vi "BlueToothOff.vi"(4 "Connected":bool, 5 "Partner Name":string, 6 "Connection":u8, 7 "NXT/EV3":T1) -> (1 "Success":bool, 2 "NXTBTPower":i8, 3 "NXT/EV3 2":T1)   [LabVIEW 2013]
uses:
  <vilib>/NXT/Subs/LVHSConnector.ctl
  <vilib>/NXT/LegoClasses/BrickReference/BrickReference.lvclass
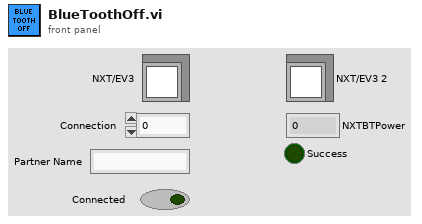
[diagram p1: front panel]
types:
  T1 = typedef "LVHSConnector.ctl" = refnum<class "BrickReference.lvclass">
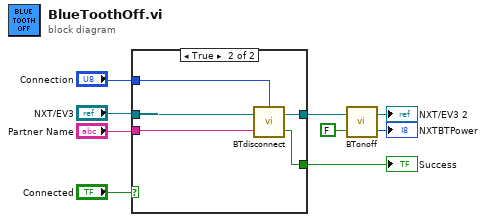
[diagram p0: block diagram]
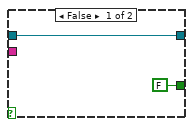
[diagram p2: hidden frame]
diagram:
  n1 = case shown="True" "Connected" {
    tunnel: "NXT/EV3" -> [w11 w16]
    tunnel: [w11 w15] -> w7
    tunnel: [FALSE ("Success") w14] -> w3
    tunnel: "Partner Name" -> [_ w13]
    tunnel: "Connection" -> [_ w12]
    frame False {
    }
    frame True {
      n2 = call <vilib>:"BTdisconnect.vi"("Partner Name"=w13, "NXT/EV3"=w16, "Connection"=w12) -> ("Success"=w14:bool, "NXT/EV3"=w15:T1)
    }
  }
  "Success" <- w3
  n3 = call <vilib>:"BTonoff.vi"("On/Off"=FALSE, "NXT/EV3"=w7) -> ("NXTBTPower"=→"NXTBTPower":i8, "NXT/EV3"=→"NXT/EV3 2":T1)  [unwired: 1 in]
